vi "Inst Configuration.vi"() -> ()   [LabVIEW 2016, in "User Interface.lvlib"]
uses:
  User Interface.lvlib
  Inst Config Command.ctl
  <vilib>/Utility/miscctls.llb/LVPointTypeDef.ctl
  VI Name.ctl
panel:
  in  "Tab Control":T1(tab)
  out "error out":errorcluster
  in  "error in (no error)":errorcluster
  in  "EXIT":bool
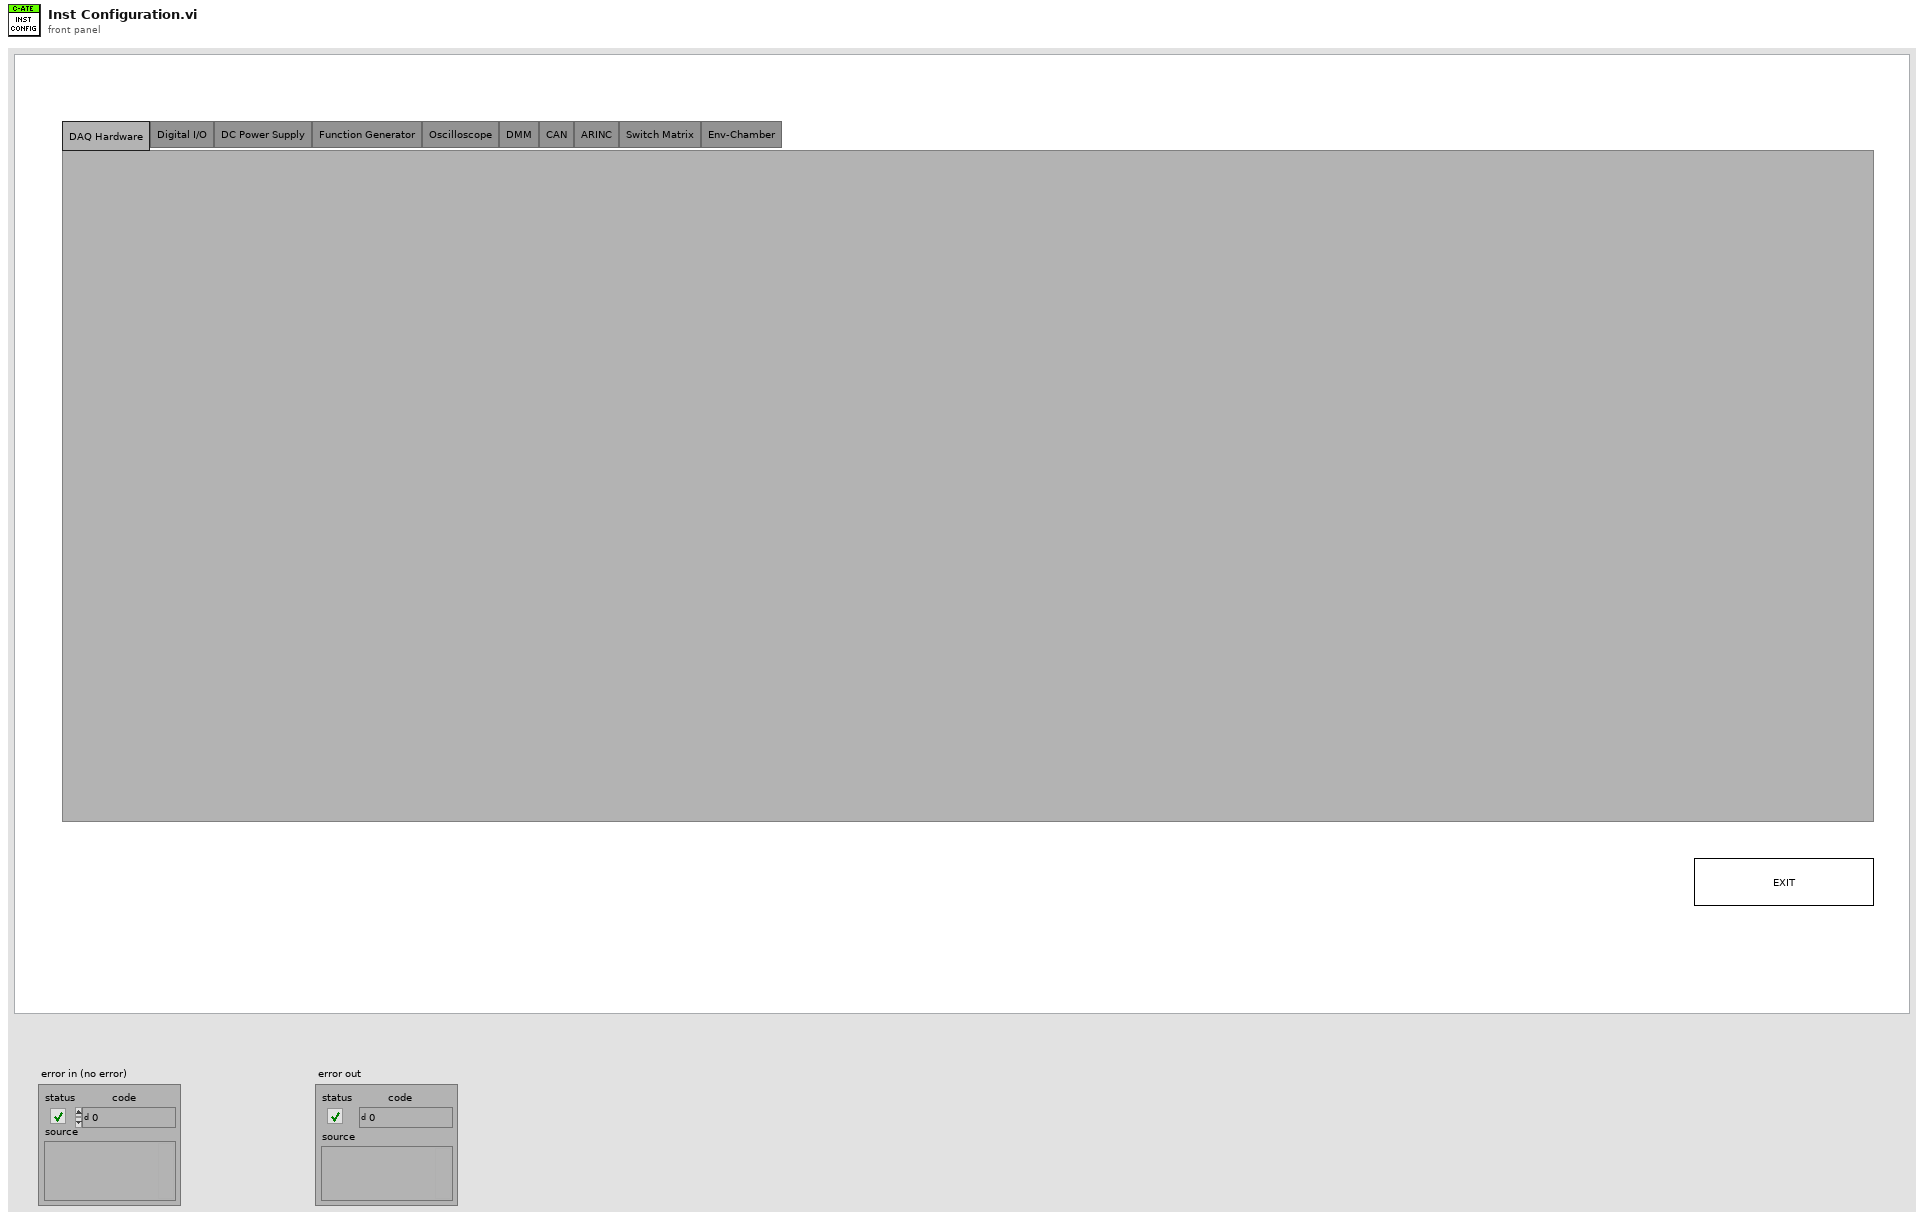
[diagram p1: front panel]
types:
  T1 = enum32{"DAQ Hardware", "Digital I/O", "DC Power Supply", "Function Generator", "Oscilloscope", "DMM", "CAN", "ARINC", "Switch Matrix", "Env-Chamber"}
  T2 = typedef "LVPointTypeDef.ctl" = cluster{"Horizontal":i16, "Vertical":i16}
  T3 = typedef "User Interface.lvlib/Inst Config Command.ctl" = enum16{"Init", "Main", "Close"}
  T4 = typedef "User Interface.lvlib/VI Name.ctl" = enum16{"Dashboard", "Maintenance", "Recipe", "Inst Configuration", "Testing", "Report"}
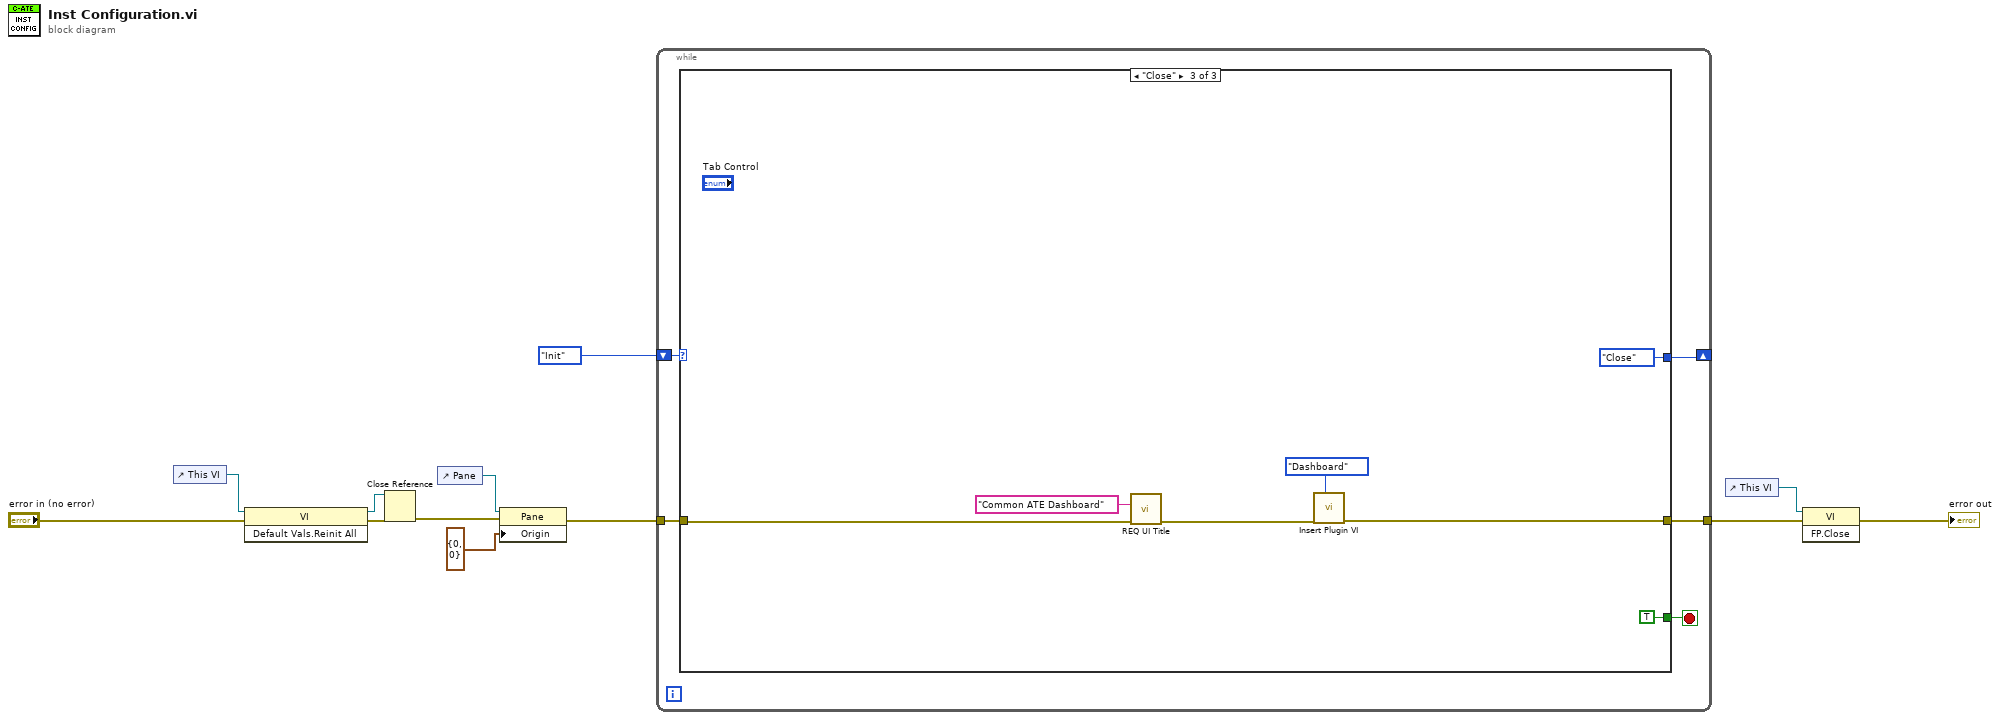
[diagram p0: block diagram]
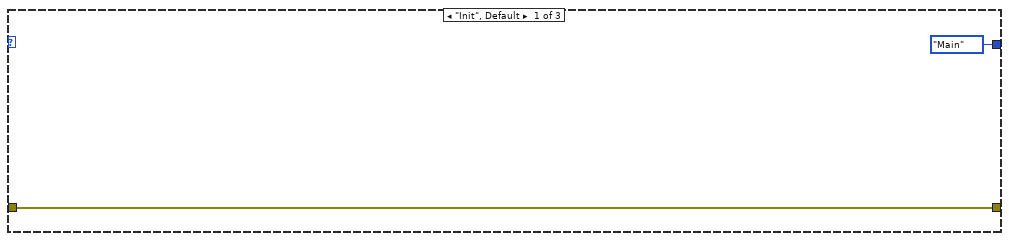
[diagram p2: hidden frame]
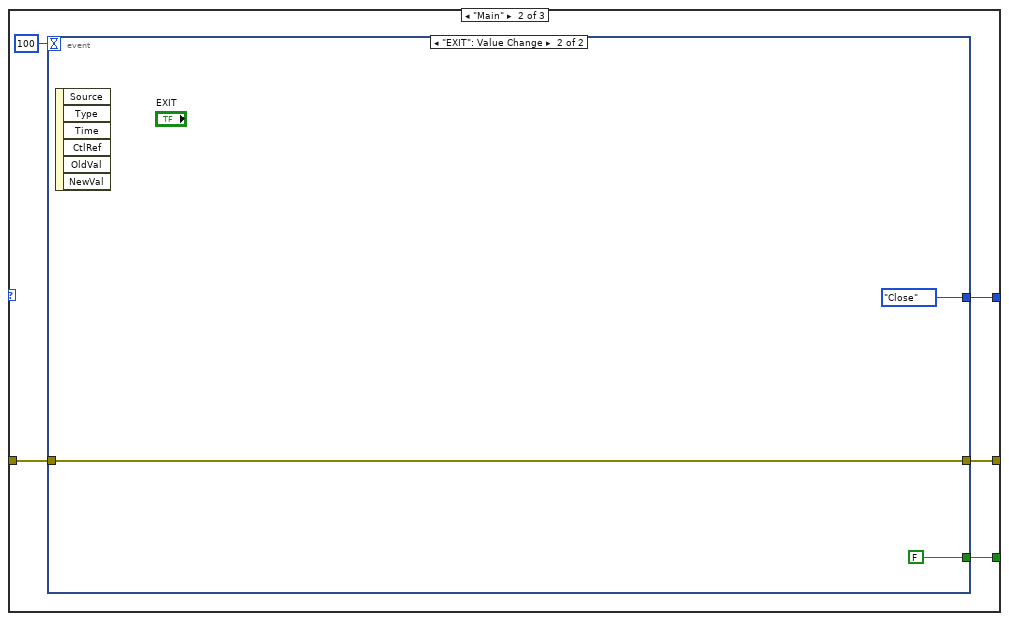
[diagram p3: hidden frame]
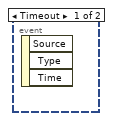
[diagram p4: hidden frame]
diagram:
  n1 = control-ref of="This VI"() -> (w5:refnum<vi>)
  n2 = invoke class="VI" method="Default Vals.Reinit All"(reference=w5, error in="error in (no error)") -> (reference out=w3:refnum<vi>, error out=w4:errorcluster)  [unwired: 1 in, 1 out]
  n3 = Close Reference(reference=w3, error in (no error)=w4) -> (error out=w1:errorcluster)
  n4 = control-ref of="Pane"() -> (w12:refnum<vi>)
  n5 = property class="Pane"(reference=w12, error in=w1, "Origin"=T2 {"Horizontal"=0, "Vertical"=0}) -> (error out=w11:errorcluster)  [unwired: 1 out]
  n6 = while {
    tunnel: w11 -> [w17]
    shift-right: [w13] -> _
    shift-left: Inst_Config_Command."Init" -> [w16]
    tunnel: [w15] -> w7
    stop <- w14 stop-if-true
    n7 = case shown="\"Close\"" w16 {
      tunnel: w17 -> [w18 w23 w29]
      tunnel: [w18 w22 w33] -> w15
      tunnel: [_ w21 TRUE] -> w14
      tunnel: [Inst_Config_Command."Main" w20 Inst_Config_Command."Close"] -> w13
      frame "Init", Default {
      }
      frame "Main" {
        n8 = event shown="[1] \"EXIT\": Value Change" {
          selector: _ -> [_ _]
          dyn-events: _ -> [_ _]
          timeout: 100 -> [_ _]
          tunnel: w23 -> [_ w27]
          tunnel: [_ w27] -> w22
          tunnel: [_ FALSE] -> w21
          tunnel: [_ Inst_Config_Command."Close"] -> w20
          event Timeout {
            n9 = event-data() -> ()  [unwired: 1 in, 3 out]
          }
          event "EXIT": Value Change {
            n10 = event-data() -> ()  [unwired: 1 in, 6 out]
          }
        }
      }
      frame "Close" {
        n11 = call "REQ UI Title.vi"("error in"=w29, "UI Title"="Common ATE Dashboard" ("ATE Title")) -> ("error out"=w28:errorcluster)  [unwired: 9 in]
        n12 = call "Insert Plugin VI.vi"("VI Name"=VI_Name."Dashboard", "error in (no error)"=w28) -> ("error out"=w33:errorcluster)  [unwired: 9 in]
      }
    }
  }
  n13 = control-ref of="This VI"() -> (w8:refnum<vi>)
  n14 = invoke class="VI" method="FP.Close"(reference=w8, error in=w7) -> (error out=→"error out":errorcluster)  [unwired: 1 in, 2 out]
